vi "read_write2.vi"() -> ()   [LabVIEW 2014]
panel:
  in  "Description":string
  out "Filename":path
  in  "Function":u16(ring) items=["Sinh", "Cosh", "Tan", "Cos", "Sin"]
  out "YArray":dbl[](array[numeric])
  out "XArray":dbl[](array[numeric])
  out "XSteps":dbl
  in  "XEnd":dbl
  in  "XRes":dbl
  in  "XStart":dbl
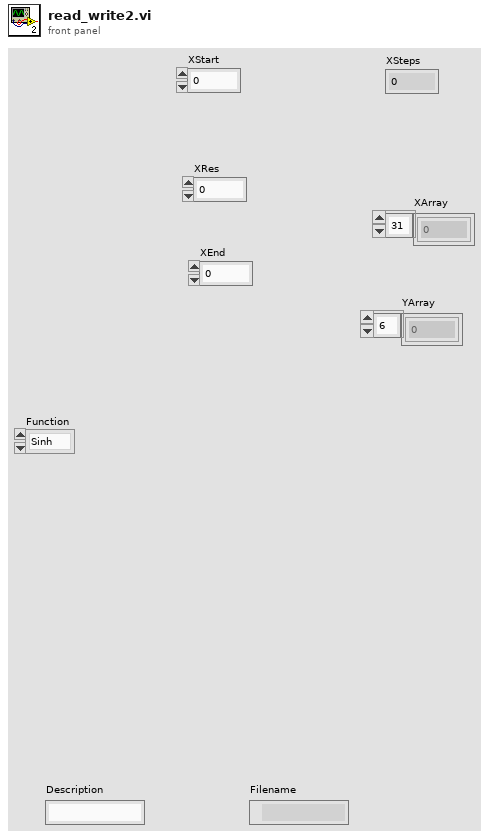
[diagram p1: front panel]
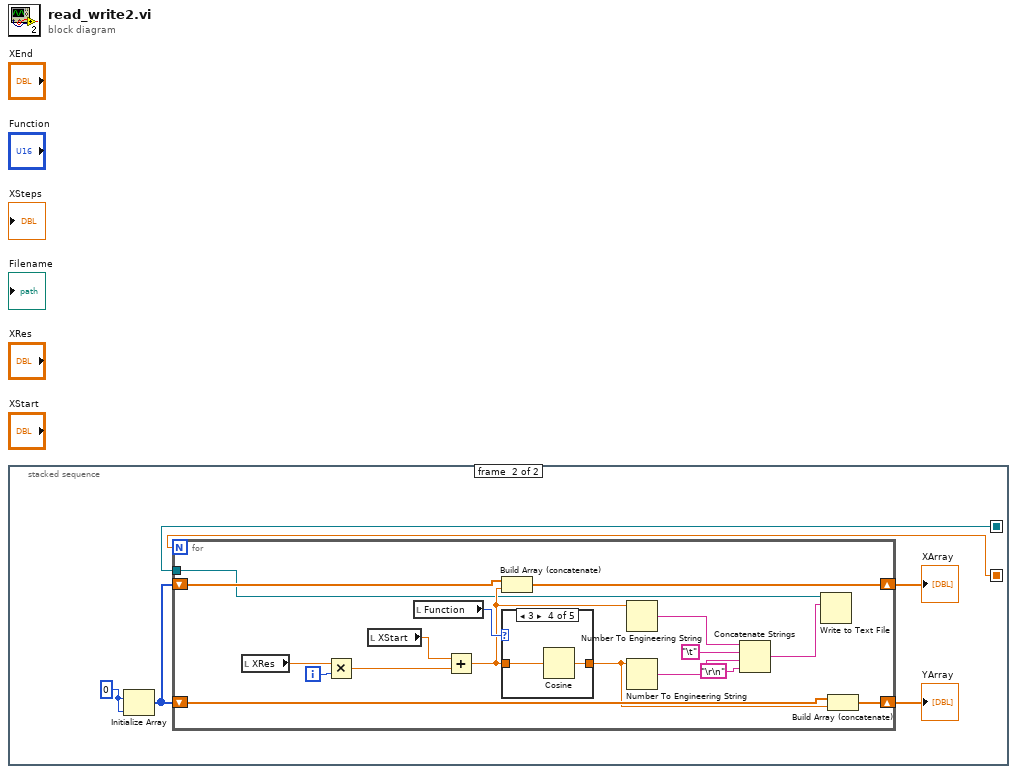
[diagram p0: block diagram]
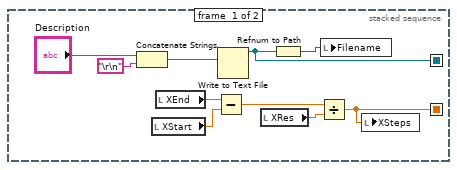
[diagram p2: hidden frame]
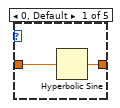
[diagram p3: hidden frame]
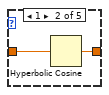
[diagram p4: hidden frame]
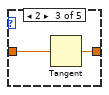
[diagram p5: hidden frame]
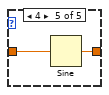
[diagram p6: hidden frame]
diagram:
  n1 = stacked-sequence {
    seq-local: [w6 _] -> [_ w16]
    seq-local: [w1 _] -> [_ w11]
    frame #0 {
      n2 = Concatenate Strings("Description", "\r\n") -> (w3:string)
      n3 = local read "XStart"() -> (w9:dbl)
      n4 = local read "XEnd"() -> (w10:dbl)
      n5 = Subtract(x=w10, y=w9) -> (x-y=w8:dbl)
      n6 = Write to Text File(text=w3) -> (refnum out=w1:refnum<file>)  [unwired: 3 in, 2 out]
      n7 = local read "XRes"() -> (w7:dbl)
      n8 = Refnum to Path(1:w1) -> (0:w2:path)
      n9 = Divide(x=w8, y=w7) -> (x/y=w6:dbl)
      n10 = local write "Filename"(w2) -> ()
      n11 = local write "XSteps"(w6) -> ()
    }
    frame #1 {
      w15 = 0
      n12 = Initialize Array(w15, w15) -> (w12:i32[])
      n13 = for {
        N: w16 -> [_]
        shift-right: [w28] -> w14
        shift-left: w12 -> [w29]
        shift-right: [w25] -> w13
        shift-left: w12 -> [w26]
        tunnel: w11 -> [w17]
        i -> [w32]
        n14 = local read "XRes"() -> (w33:dbl)
        n15 = Multiply(x=w33, y=w32) -> (x*y=w30:dbl)
        n16 = local read "XStart"() -> (w31:dbl)
        n17 = local read "Function"() -> (w27:u16)
        n18 = Add(x=w31, y=w30) -> (x+y=w24:dbl)
        n19 = Build Array (concatenate)(w29, w24) -> (w28:dbl[])
        n20 = case shown="3" w27 {
          tunnel: w24 -> [w35 w37 w39 w41 w43]
          tunnel: [w34 w36 w38 w40 w42] -> w23
          frame 0, Default {
            n21 = Hyperbolic Sine(1:w35) -> (0:w34:dbl)
          }
          frame 1 {
            n22 = Hyperbolic Cosine(1:w37) -> (0:w36:dbl)
          }
          frame 2 {
            n23 = Tangent(1:w39) -> (0:w38:dbl)
          }
          frame 3 {
            n24 = Cosine(x=w41) -> (cos(x)=w40:dbl)
          }
          frame 4 {
            n25 = Sine(x=w43) -> (sin(x)=w42:dbl)
          }
        }
        n26 = Number To Engineering String(4:w24) -> (0:w22:string)  [unwired: 3 in]
        n27 = Number To Engineering String(4:w23) -> (0:w20:string)  [unwired: 3 in]
        n28 = Concatenate Strings(w22, "\t", w20, "\r\n") -> (w18:string)
        n29 = Write to Text File(file (use dialog)=w17, text=w18) -> ()  [unwired: 2 in, 3 out]
        n30 = Build Array (concatenate)(w26, w23) -> (w25:dbl[])
      }
      "XArray" <- w14
      "YArray" <- w13
    }
  }
